vi "Lab-Hub.vi"() -> ()   [LabVIEW 2017]
panel:
  in  "WT Control":bool=TRUE
  in  "Measurement Software":bool
  in  "Move Traverse":bool
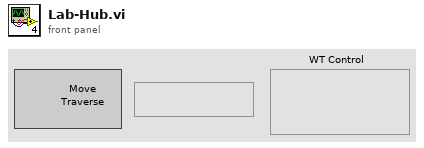
[diagram p1: front panel]
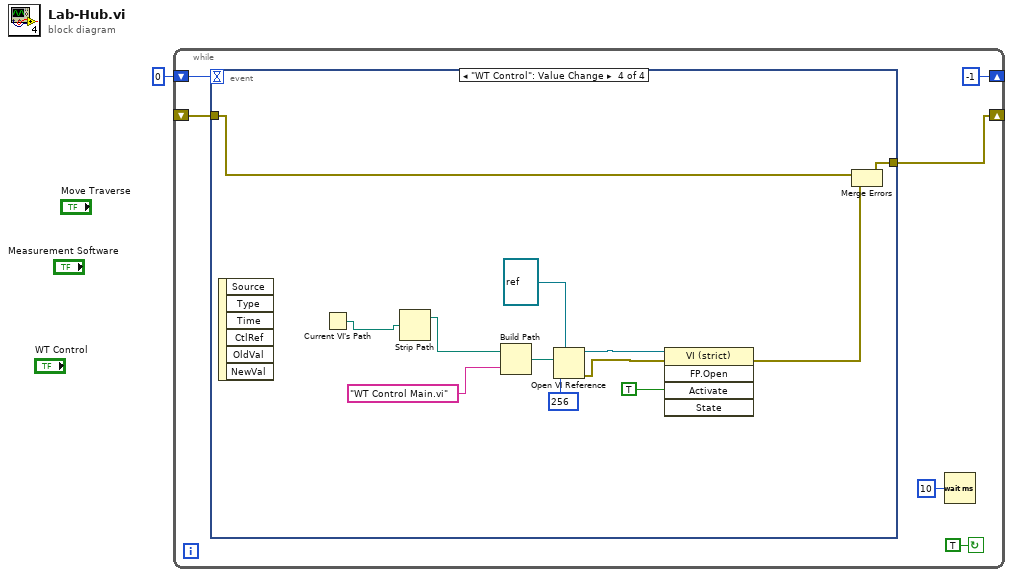
[diagram p0: block diagram]
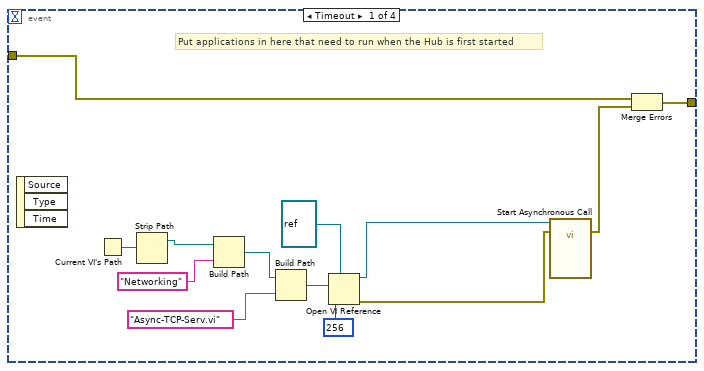
[diagram p2: hidden frame]
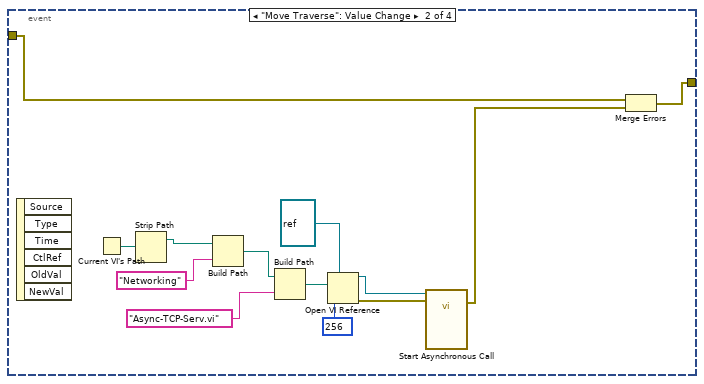
[diagram p3: hidden frame]
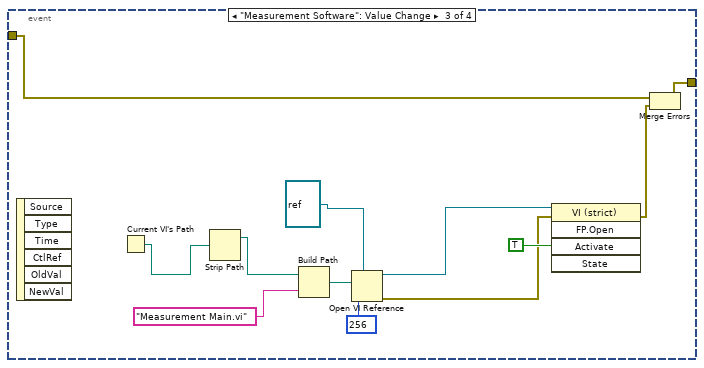
[diagram p4: hidden frame]
diagram:
  n1 = while {
    shift-right: [-1] -> _
    shift-left: 0 -> [w6]
    shift-right: [w3] -> _
    shift-left: _ -> [w2]
    stop <- TRUE continue-if-true
    n2 = event shown="[3] \"WT Control\": Value Change" {
      selector: _ -> [_ _ _ _]
      dyn-events: _ -> [_ _ _ _]
      timeout: w6 -> [_ _ _ _]
      tunnel: [w9 w25 w41 w53] -> w3
      tunnel: w2 -> [w8 w24 w42 w54]
      event Timeout {
        # "Put applications in here that need to run when the Hub is first started"
        n3 = event-data() -> ()  [unwired: 1 in, 3 out]
        n4 = Current VI's Path() -> (path=w20:path)
        n5 = Strip Path(path=w20) -> (stripped path=w16:path)  [unwired: 1 out]
        n6 = Build Path(base path=w16, name or relative path="Networking") -> (appended path=w15:path)
        n7 = Build Path(base path=w15, name or relative path="Async-TCP-Serv.vi") -> (appended path=w18:path)
        n8 = Open VI Reference(type specifier VI Refnum (for type only)=refnum<vi> refnum, vi path=w18, options=256) -> (vi reference=w12:refnum<vi>, error out=w11:errorcluster)  [unwired: 3 in]
        n9 = call-by-ref "Start Asynchronous Call"(reference=w12, error in=w11) -> (error out=w10:errorcluster)  [unwired: 12 in, 1 out]
        n10 = Merge Errors(w8, w10) -> (w9:errorcluster)
      }
      event "Move Traverse": Value Change {
        n11 = event-data() -> ()  [unwired: 1 in, 6 out]
        n12 = Current VI's Path() -> (path=w33:path)
        n13 = Strip Path(path=w33) -> (stripped path=w29:path)  [unwired: 1 out]
        n14 = Build Path(base path=w29, name or relative path="Networking") -> (appended path=w28:path)
        n15 = Build Path(base path=w28, name or relative path="Async-TCP-Serv.vi") -> (appended path=w31:path)
        n16 = Open VI Reference(type specifier VI Refnum (for type only)=refnum<vi> refnum, vi path=w31, options=256) -> (vi reference=w22:refnum<vi>, error out=w26:errorcluster)  [unwired: 3 in]
        n17 = call-by-ref "Start Asynchronous Call"(reference=w22, error in=w26) -> (error out=w23:errorcluster)  [unwired: 12 in, 1 out]
        n18 = Merge Errors(w24, w23) -> (w25:errorcluster)
      }
      event "Measurement Software": Value Change {
        n19 = event-data() -> ()  [unwired: 1 in, 6 out]
        n20 = Current VI's Path() -> (path=w39:path)
        n21 = Strip Path(path=w39) -> (stripped path=w38:path)  [unwired: 1 out]
        n22 = Build Path(base path=w38, name or relative path="Measurement Main.vi") -> (appended path=w44:path)
        n23 = Open VI Reference(type specifier VI Refnum (for type only)=refnum<vi> refnum, vi path=w44, options=256) -> (vi reference=w36:refnum<vi>, error out=w35:errorcluster)  [unwired: 3 in]
        n24 = invoke class="VI (strict)" method="FP.Open"(reference=w36, error in=w35, "Activate"=TRUE ("Activate?")) -> (error out=w34:errorcluster)  [unwired: 2 in, 4 out]
        n25 = Merge Errors(w42, w34) -> (w41:errorcluster)
      }
      event "WT Control": Value Change {
        n26 = event-data() -> ()  [unwired: 1 in, 6 out]
        n27 = Current VI's Path() -> (path=w51:path)
        n28 = Strip Path(path=w51) -> (stripped path=w50:path)  [unwired: 1 out]
        n29 = Build Path(base path=w50, name or relative path="WT Control Main.vi") -> (appended path=w56:path)
        n30 = Open VI Reference(type specifier VI Refnum (for type only)=refnum<vi> refnum, vi path=w56, options=256) -> (vi reference=w49:refnum<vi>, error out=w48:errorcluster)  [unwired: 3 in]
        n31 = invoke class="VI (strict)" method="FP.Open"(reference=w49, error in=w48, "Activate"=TRUE ("Activate?")) -> (error out=w46:errorcluster)  [unwired: 2 in, 4 out]
        n32 = Merge Errors(w54, w46) -> (w53:errorcluster)
      }
    }
    n33 = Wait (ms)(milliseconds to wait=u32 10) -> ()  [unwired: 1 out]
  }
